vi "Unregister.vi"(8 "error in":errorcluster, 11 "Win32 Event in":refnum<class "Win32 Event.lvclass">) -> (0 "error out":errorcluster, 3 "Win32 Event out":refnum<class "Win32 Event.lvclass">)   [LabVIEW 2019, in "PCANBasic.lvlib" / "Win32 Event.lvclass"]
uses:
  Win32 Event.lvclass
  TPCANHandle.ctl
  Win32 Event.lvclass/Win32 Event.ctl
  PCANBasic.lvlib
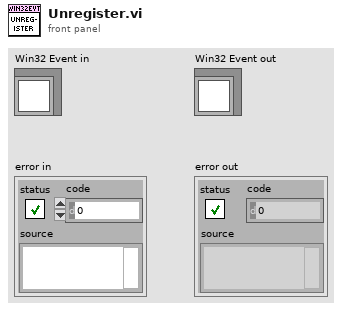
[diagram p1: front panel]
types:
  T1 = typedef "PCANBasic.lvlib/TPCANHandle.ctl" = u16
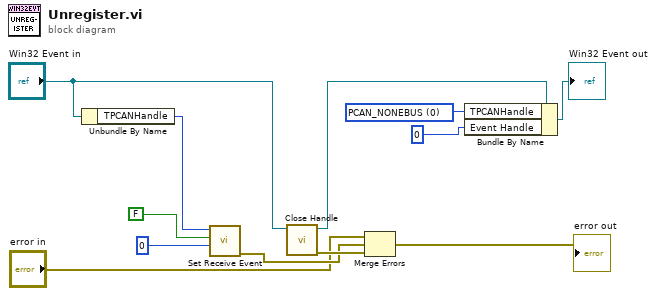
[diagram p0: block diagram]
diagram:
  w2 = T1 0 items=["PCAN_NONEBUS"=0, "PCAN_USBBUS1"=81, "PCAN_USBBUS2"=82, "PCAN_USBBUS3"=83, "PCAN_USBBUS4"=84, "PCAN_USBBUS5"=85, "PCAN_USBBUS6"=86, "PCAN_USBBUS7"=87, "PCAN_USBBUS8"=88, "PCAN_USBBUS9"=1289, "PCAN_USBBUS10"=1290, "PCAN_USBBUS11"=1291, "PCAN_USBBUS12"=1292, "PCAN_USBBUS13"=1293, "PCAN_USBBUS14"=1294, "PCAN_USBBUS15"=1295, "PCAN_USBBUS16"=1296] ("TPCANHandle")
  n1 = Unbundle By Name("Win32 Event in") -> ("TPCANHandle"=w12:T1)
  n2 = call "Set Receive Event.vi"("Event Handle"=u64 0, "Enable"=FALSE, "TPCANHandle in"=w12) -> ("error out"=w6:errorcluster)  [unwired: 6 in, 2 out]
  n3 = call "Close Handle.vi"("Win32 Event in"="Win32 Event in") -> ("error out"=w8:errorcluster, "Win32 Event out"=w4:refnum<class "Win32 Event.lvclass">)  [unwired: 9 in]
  n4 = Merge Errors("error in", w6, w8) -> (→"error out":errorcluster)
  n5 = Bundle By Name(cluster=w4, "TPCANHandle"=w2, "Event Handle"=u64 0) -> (→"Win32 Event out":refnum<class "Win32 Event.lvclass">)
